vi "p1.vi"() -> ()   [LabVIEW 2023, in "d15.lvlib"]
uses:
  d15.lvlib
  AOC/AOC.lvlib
panel:
  in  "Example":string="rn=1,cm-,qp=3,cm=2,qp-,pc=4,ot=9,ab=5,pc-,pc=6,ot=7"
  in  "Example":bool
  out "Answer":u64=4737443
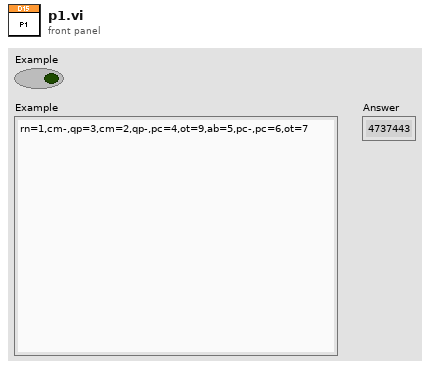
[diagram p1: front panel]
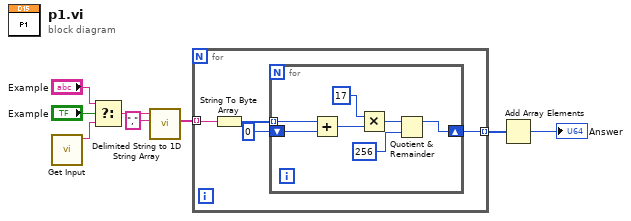
[diagram p0: block diagram]
diagram:
  n1 = call "Get Input.vi"() -> ("Input"=w8:string)  [unwired: 11 in]
  n2 = Select(t="Example", s="Example", f=w8) -> (s? t:f=w4:string)
  n3 = call <vilib>:"Delimited String to 1D String Array.vi"("delimiter"=",", "delimited string"=w4) -> ("string array"=w5:string[])  [unwired: 9 in]
  n4 = for {
    tunnel: w5 -> [w11] mode=indexing
    tunnel: [w9] -> w2 mode=indexing
    n5 = String To Byte Array(string=w11) -> (unsigned byte array=w10:u8[])
    n6 = for {
      shift-right: [w13] -> w9
      shift-left: u64 0 -> [w19]
      tunnel: w10 -> [w18] mode=indexing
      n7 = Add(x=w18, y=w19) -> (x+y=w17:u64)
      n8 = Multiply(x=u64 17, y=w17) -> (x*y=w15:u64)
      n9 = Quotient & Remainder(x=w15, y=u64 256) -> (x-y*floor(x/y)=w13:u64)  [unwired: 1 out]
    }
  }
  n10 = Add Array Elements(numeric array=w2) -> (sum=→"Answer":u64)
